vi "Read IExporter.vi"(11 "CDependencyInspection in":refnum<class "CDependencyInspection.lvclass">) -> (2 "IExporter":refnum<class "IExporter.lvclass">, 3 "CDependencyInspection out":refnum<class "CDependencyInspection.lvclass">)   [LabVIEW 2020, in "DependencyInspection.lvlib" / "CDependencyInspection.lvclass"]
uses:
  CDependencyInspection.lvclass
  ExtensionInterfaces/IExporter/IExporter.lvclass
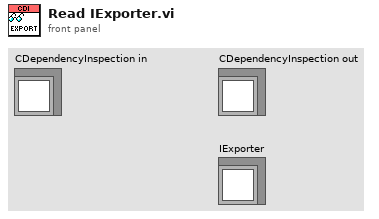
[diagram p1: front panel]
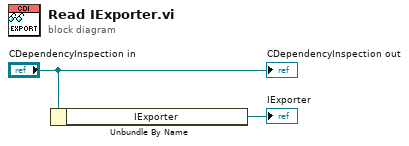
[diagram p0: block diagram]
diagram:
  n1 = Unbundle By Name("CDependencyInspection in") -> ("IExporter"=→"IExporter":refnum<class "IExporter.lvclass">)
  "CDependencyInspection out" <- "CDependencyInspection in"
